vi "Configure Channel Equation.vi"(5 "Enable Differential (T: Enable)":bool=TRUE, 7 "Enable Comm (T: Enable)":bool=TRUE, 8 "error in (no error)":errorcluster, 9 "Skew (1 ms)":dbl=0.001, 10 "Channel (1: Channel 1)":i32(ring)=1 items=["Channel 1"=1, "Channel 2"=2, "Channel 3"=3, "Channel 4"=4], 11 "VISA resource name":refnum<visa-resource-name>) -> (0 "error out":errorcluster, 3 "VISA resource name out":refnum<visa-resource-name>)   [LabVIEW 2013, in "Agilent 90000 Series.lvlib"]
doc: "Configures the equation of the oscilloscope for the specified channel. \n\n<B>Note:</B>\nThis VI is only valid for 9000 series."
uses:
  Agilent 90000 Series.lvlib
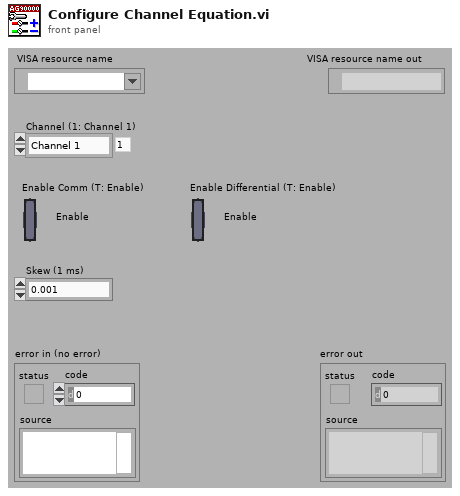
[diagram p1: front panel]
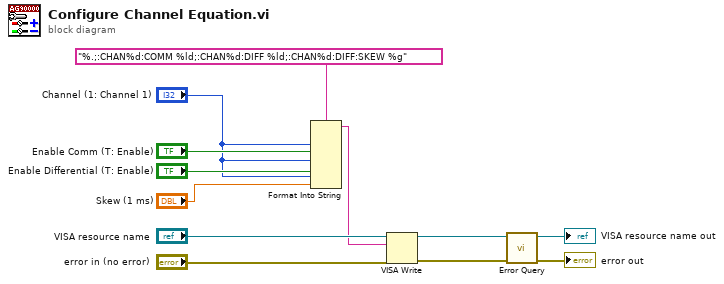
[diagram p0: block diagram]
diagram:
  n1 = Format Into String(format string="%.;:CHAN%d:COMM %ld;:CHAN%d:DIFF %ld;:CHAN%d:DIFF:SKEW %g", "Channel (1: Channel 1)", "Enable Comm (T: Enable)", "Channel (1: Channel 1)", "Enable Differential (T: Enable)", "Channel (1: Channel 1)", "Skew (1 ms)") -> (resulting string=w5:string)  [unwired: 2 in, 1 out]
  n2 = VISA Write(VISA resource name="VISA resource name", write buffer=w5, error in (no error)="error in (no error)") -> (VISA resource name out=w4:refnum<visa-resource-name>, error out=w3:errorcluster)  [unwired: 1 out]
  n3 = call "Error Query.vi"("error in (no error)"=w3, "VISA resource name"=w4) -> ("error out"=→"error out":errorcluster, "VISA resource name out"=→"VISA resource name out":refnum<visa-resource-name>)  [unwired: 8 out]
